vi "All Meta.vi"(8 "error in (no error)":errorcluster, 11 "Config Element In":refnum<class "Config Element.lvclass">) -> (0 "error out":errorcluster, 2 "Meta Data":T1[](array[typedef]), 3 "Config Element":refnum<class "Config Element.lvclass">)   [LabVIEW 2020, in "CDM-Config.lvlib" / "Config Element.lvclass"]
uses:
  Config Element.lvclass
  Meta Data.ctl
  Config Element.lvclass/Config Element.ctl
  CDM-Config.lvlib
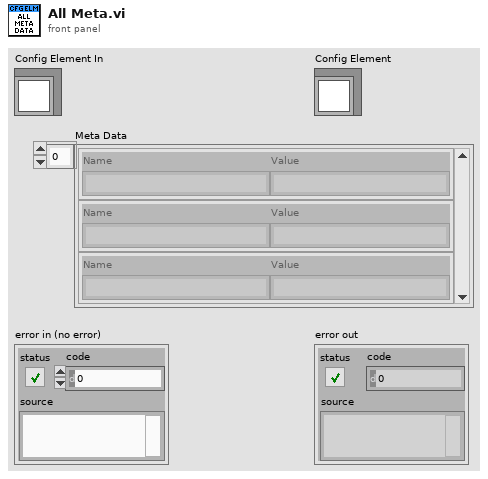
[diagram p1: front panel]
types:
  T1 = typedef "CDM-Config.lvlib/Meta Data.ctl" = cluster{"Name":string, "Value":string}
  T2 = typedef "CDM-Config.lvlib/Config Element.lvclass/Ref Data.ctl" = cluster{"Config Element":T3, "Node Info":T4, "Owner":refnum<class>, "Changed":bool}
  T3 = typedef "CDM-Config.lvlib/Config Element.ctl" = cluster{"Hierarchy":string[], "Value":string, "Meta Data":T1[]}
  T4 = typedef "CDM-Config.lvlib/Node Info.ctl" = cluster{"Index":i32, "Parent":i32, "Children":i32[]}
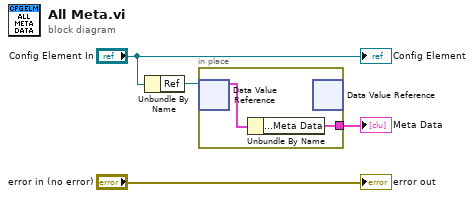
[diagram p0: block diagram]
diagram:
  n1 = Unbundle By Name("Config Element In") -> ("Ref"=w4:refnum<data-value>)
  n2 = in-place {
    in-place-border: [w5] -> w2
    n3 = in-place-dvr #1(w4) -> (w6:T2)  [unwired: 1 out]
    n4 = Unbundle By Name(w6) -> ("Config Element.Meta Data"=w5:T1[])
    n5 = in-place-dvr #1() -> ()  [unwired: 1 in, 2 out]
  }
  "Meta Data" <- w2
  "Config Element" <- "Config Element In"
  "error out" <- "error in (no error)"
